vi "Object data correction and extraction.vi"(5 "Cmd":string="(ta,to,x,y,z,0,0,o)", 6 "Sorted array":dbl[][](array[numeric]), 7 "Object number of interest":i32, 8 "y":dbl=406.2 format="%#_13g", 9 "x":dbl=-35.0 format="%#_13g") -> (0 "Corrected Object orientation":dbl, 1 "Object CoM X":dbl, 2 "Object CoM Y":dbl, 3 "Obejct length":dbl, 4 "Assignment Coordinates":string)   [LabVIEW 2024]
doc: "Takes the object data array and a insect number and output the coordinates, length and orientation of the chosen object"
panel:
  out "Angle in Range":bool
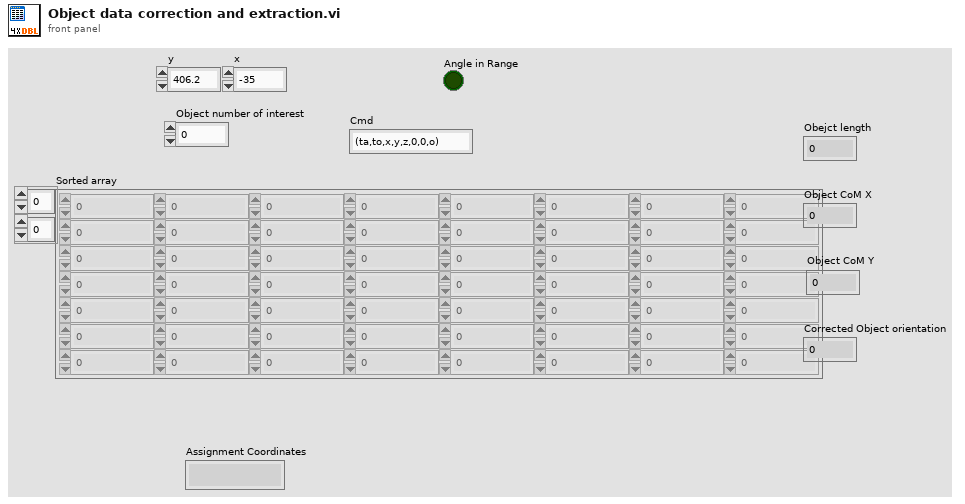
[diagram p1: front panel]
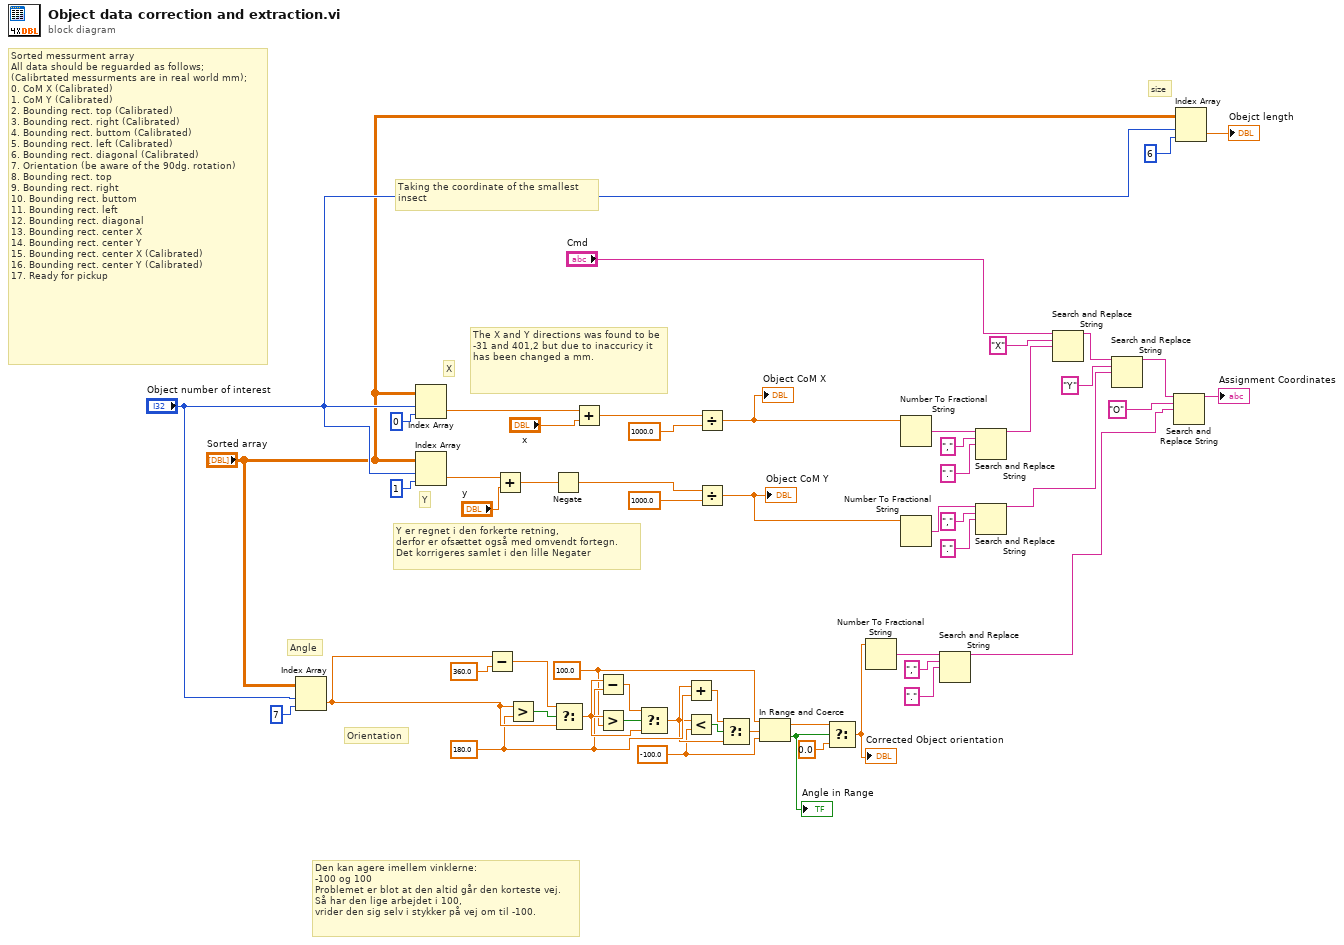
[diagram p0: block diagram]
diagram:
  w16 = -100.0 ("y")
  w20 = 180.0 ("y")
  w17 = 100.0 ("y")
  # "Sorted messurment array\nAll data should be reguarded as follows;\n(Calibrtated messurments are in real world mm);\n0. CoM X (Calibrated)\n1. CoM Y (Calibrated)\n2. Bounding rect. top (Calibrated)\n3. Bounding rect. right (Calibrated)\n4. Bounding rect. buttom (Calibrated)\n5. Bounding rect. left (Calibrated)\n6. Bounding rect. diagonal (Calibrated)\n7. Orientation (be aware of the 90dg. rotation)\n8. Bounding rect. top\n9. Bounding rect. right\n10. Bounding rect. buttom\n11. Bounding rect. left\n12. Bounding rect. diagonal\n13. Bounding rect. center X\n14. Bounding rect. center Y\n15. Bounding rect. center X (Calibrated)\n16. Bounding rect. center Y (Calibrated)\n17. Ready for pickup"
  # "The X and Y directions was found to be -31 and 401,2 but due to inaccuricy it has been changed a mm."
  # "Den kan agere imellem vinklerne:\n-100 og 100\nProblemet er blot at den altid går den korteste vej.\nSå har den lige arbejdet i 100, \nvrider den sig selv i stykker på vej om til -100."
  # "Y er regnet i den forkerte retning, \nderfor er ofsættet også med omvendt fortegn.\nDet korrigeres samlet i den lille Negater"
  # "Angle"
  # "Y"
  # "X"
  # "size"
  # "Taking the coordinate of the smallest \ninsect"
  # "Orientation"
  n1 = Index Array(array="Sorted array", index (row)="Object number of interest", index (col)=7 ("disabled index (col)")) -> (element=w23:dbl)
  n2 = Index Array(array="Sorted array", index (row)="Object number of interest", index (col)=0 ("disabled index (col)")) -> (element=w44:dbl)
  n3 = Index Array(array="Sorted array", index (row)="Object number of interest", index (col)=1 ("disabled index (col)")) -> (element=w42:dbl)
  n4 = Subtract(x=w23, y=360.0) -> (x-y=w26:dbl)
  n5 = Add(x=w42, y="y") -> (x+y=w45:dbl)
  n6 = Greater?(x=w23, y=w20) -> (0:w27:bool)
  n7 = Negate(x=w45) -> (-x=w48:dbl)
  n8 = Select(t=w26, s=w27, f=w23) -> (s? t:f=w24:dbl)
  n9 = Add(x=w44, y="x") -> (x+y=w49:dbl)
  n10 = Subtract(x=w24, y=w20) -> (x-y=w28:dbl)
  n11 = Greater?(x=w24, y=w17) -> (0:w29:bool)
  n12 = Select(t=w28, s=w29, f=w24) -> (s? t:f=w18:dbl)
  n13 = Add(x=w18, y=w20) -> (x+y=w19:dbl)
  n14 = Less?(x=w18, y=w16) -> (x < y?=w21:bool)
  n15 = Divide(x=w49, y=1000.0) -> (x/y=w31:dbl)
  "Object CoM X" <- w31
  n16 = Divide(x=w48, y=1000.0) -> (x/y=w30:dbl)
  "Object CoM Y" <- w30
  n17 = Select(t=w19, s=w21, f=w18) -> (s? t:f=w22:dbl)
  n18 = In Range and Coerce(upper limit=w17, x=w22, lower limit=w16) -> (coerced(x)=w14:dbl, In Range?=w15:bool)
  "Angle in Range" <- w15
  n19 = Select(t=w14, s=w15, f=0.0) -> (s? t:f=w13:dbl)
  "Corrected Object orientation" <- w13
  n20 = Number To Fractional String(number=w13) -> (F-format string=w33:string)  [unwired: 3 in]
  n21 = Number To Fractional String(number=w31) -> (F-format string=w32:string)  [unwired: 3 in]
  n22 = Number To Fractional String(number=w30) -> (F-format string=w36:string)  [unwired: 3 in]
  n23 = Search and Replace String(input string=w33, search string=",", replace string="." ("replace string (\"\")")) -> (result string=w3:string)  [unwired: 5 in, 3 out]
  n24 = Search and Replace String(input string=w32, search string=",", replace string="." ("replace string (\"\")")) -> (result string=w9:string)  [unwired: 5 in, 3 out]
  n25 = Search and Replace String(input string=w36, search string=",", replace string="." ("replace string (\"\")")) -> (result string=w7:string)  [unwired: 5 in, 3 out]
  n26 = Search and Replace String(input string="Cmd", search string="X", replace string=w9) -> (result string=w6:string)  [unwired: 5 in, 3 out]
  n27 = Search and Replace String(input string=w6, search string="Y", replace string=w7) -> (result string=w5:string)  [unwired: 5 in, 3 out]
  n28 = Search and Replace String(input string=w5, search string="O" ("replace string (\"\")"), replace string=w3) -> (result string=→"Assignment Coordinates":string)  [unwired: 5 in, 3 out]
  n29 = Index Array(array="Sorted array", index (row)="Object number of interest", index (col)=6 ("disabled index (col)")) -> (element=→"Obejct length":dbl)
